vi "CameraSettingsCheck.vi"() -> ()   [LabVIEW 2017]
uses:
  <vilib>/userdefined/High Color/IMAQdx.ctl
panel:
  out "Contrast":dbl
  out "Brightness":i64
  in  "stop":bool
  out "All Edges Found":bool
  out "Session Out":T1
  in  "error in":errorcluster
  in  "Session In":T1
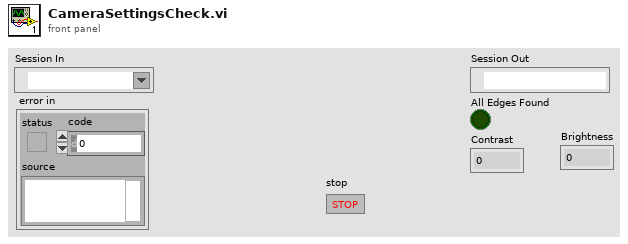
[diagram p1: front panel]
types:
  T1 = typedef "IMAQdx.ctl" = refnum<k21>
  T2 = typedef "IMAQ Coordinate System" = cluster{"Reference System":cluster{"Origin":cluster{"X":sgl, "Y":sgl}, "Angle (deg)":sgl, "Axis Reference":u32}, "Measurement System":cluster{"Origin":cluster{"X":sgl, "Y":sgl}, "Angle (deg)":sgl, "Axis Reference":u32}}
  T3 = typedef "IMAQ Image.ctl" = refnum<image>
  T4 = cluster{"Point1 (Pixels)":cluster{"X":sgl, "Y":sgl}, "Point2 (Pixels)":cluster{"X":sgl, "Y":sgl}, "Point1 (Real-World)":cluster{"X":sgl, "Y":sgl}, "Point2 (Real-World)":cluster{"X":sgl, "Y":sgl}, "Angle (Pixel)":dbl, "Angle (Real-World)":dbl, "Score":dbl, "Straightness":dbl, "Average SNR (db)":dbl, "Calibration Valid":bool}[]
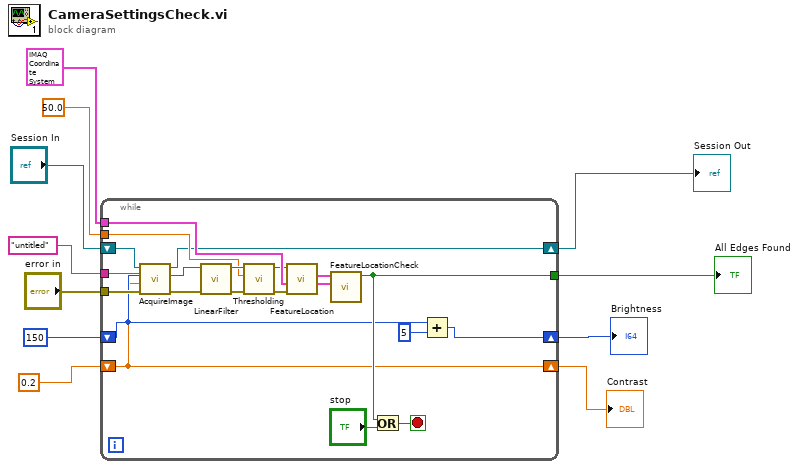
[diagram p0: block diagram]
diagram:
  n1 = while {
    tunnel: T2 {"Reference System"={"Origin"={"X"=0.0, "Y"=0.0}, "Angle (deg)"=0.0, "Axis Reference"=0}, "Measurement System"={"Origin"={"X"=0.0, "Y"=0.0}, "Angle (deg)"=0.0, "Axis Reference"=0}} ("Coordinate System") -> [w32]
    tunnel: sgl 50.0 ("Threshold Value") -> [w29]
    tunnel: "error in" -> [w23]
    tunnel: "untitled" ("Image Name") -> [w21]
    shift-right: [w22] -> w5
    shift-left: "Session In" -> [w24]
    tunnel: [w17] -> w3
    shift-right: [w13] -> w2
    shift-left: i64 150 ("Brightness") -> [w15]
    shift-right: [w12] -> w1
    shift-left: 0.2 ("Contrast") -> [w12]
    stop <- w16 stop-if-true
    n2 = call "AcquireImage.vi"("Image Name"=w21, "error in"=w23, "Contrast"=w12, "Brightness"=w15, "Session In"=w24) -> ("error out"=w19:errorcluster, "Image"=w20:T3, "Session Out"=w22:T1)  [unwired: 3 in]
    n3 = call "LinearFilter.vi"("error in (no error)"=w19, "Image Src"=w20) -> ("error out"=w30:errorcluster, "Image"=w31:T3)  [unwired: 8 in]
    n4 = call "Thresholding.vi"("error in (no error)"=w30, "Threshold Value"=w29, "Image Src"=w31) -> ("error out"=w27:errorcluster, "Image"=w28:T3)  [unwired: 7 in]
    n5 = call "FeatureLocation.vi"("error in (no error)"=w27, "Coordinate System"=w32, "Image"=w28) -> ("Vertical Edges"=w25:T4, "Horizontal Edges"=w26:T4)  [unwired: 3 in, 4 out]
    n6 = call "FeatureLocationCheck.vi"("Vertical Edges"=w25, "Horizontal Edges"=w26) -> ("All Edges Found"=w17:bool)  [unwired: 9 in]
    n7 = Or(x=w17, y="stop") -> (x .or. y?=w16:bool)
    n8 = Add(x=w15, y=i64 5) -> (x+y=w13:i64)
  }
  "Session Out" <- w5
  "All Edges Found" <- w3
  "Brightness" <- w2
  "Contrast" <- w1
